vi "create sound paths.vi"() -> (3 "Sound Paths":T1)   [LabVIEW 2017]
uses:
  controls/sound paths.ctl
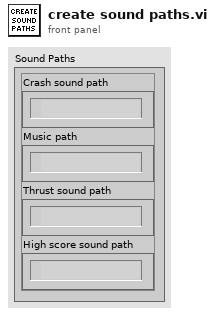
[diagram p1: front panel]
types:
  T1 = typedef "Sound Paths.ctl" = cluster{"Crash sound path":path, "Music path":path, "Thrust sound path":path, "High score sound path":path}
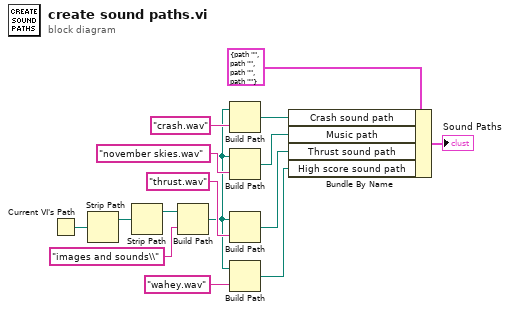
[diagram p0: block diagram]
diagram:
  n1 = Current VI's Path() -> (path=w10:path)
  n2 = Strip Path(path=w10) -> (stripped path=w11:path)  [unwired: 1 out]
  n3 = Strip Path(path=w11) -> (stripped path=w3:path)  [unwired: 1 out]
  n4 = Build Path(base path=w3, name or relative path="images and sounds\\") -> (appended path=w1:path)
  n5 = Build Path(base path=w1, name or relative path="crash.wav") -> (appended path=w8:path)
  n6 = Build Path(base path=w1, name or relative path="november skies.wav") -> (appended path=w7:path)
  n7 = Build Path(base path=w1, name or relative path="thrust.wav") -> (appended path=w6:path)
  n8 = Build Path(base path=w1, name or relative path="wahey.wav") -> (appended path=w5:path)
  n9 = Bundle By Name(cluster=T1 {"Crash sound path"=path "", "Music path"=path "", "Thrust sound path"=path "", "High score sound path"=path ""} ("Sound Paths"), "Crash sound path"=w8, "Music path"=w7, "Thrust sound path"=w6, "High score sound path"=w5) -> (→"Sound Paths":T1)
